vi "Registers in Data Clock.vi"(0 "register instruction":T6, 5 "config.resources":T4, 7 "time.resources":T3) -> (4 "read completion out":T5, 14 "ready for input":bool)   [LabVIEW 2020]
doc: "Sets/gets the configuration values for the instrument design libraries by connecting them to the Register Bus in the data clock domain.\n\n<B>Input Parameters</B>\n\n<B>register instruction</B> is the register bus instruction to execute.\n\n<B>config.resources</B> are references to the configuration registers.\n\n<B>Output Parameters</B>\n\n<B>read completion out</B> is the output of the last executed register instruction.\n\n<B>ready for input</B> is a flow control signal that indicates whether the Registers VI is ready to accept a new instruction."
uses:
  <instrlib>/_niInstr/Register Bus/v1/FPGA/Public/Register Instruction.ctl
  <instrlib>/_niInstr/Register Bus/v1/FPGA/Public/Read Completion.ctl
  <instrlib>/niUsrpRio/Time/v1/FPGA/Private/Time Resources.ctl
  <instrlib>/niUsrpRio/Time/v1/FPGA/Private/Future Event Resources.ctl
  <instrlib>/niUsrpRio/Config/v1/Shared/Subsystem ID.ctl
  <instrlib>/_niInstr/Register Bus/v1/FPGA/Private/Mux/Read Completion Mux (5 inputs).vi
  <instrlib>/_niInstr/Register Bus/v1/FPGA/niInstr Register Bus v1 FPGA.lvlib
  <instrlib>/niUsrpRio/Config/v1/FPGA/niUsrpRio Config v1 FPGA.lvlib
  <instrlib>/niUsrpRio/Config/v1/Shared/niUsrpRio Config v1 Shared.lvlib
  <instrlib>/niUsrpRio/Instruction Synchronizer/v1/FPGA/niUsrpRio Instruction Synchronizer v1 FPGA.lvlib
  <instrlib>/niUsrpRio/Time/v1/FPGA/niUsrpRio Time v1 FPGA.lvlib
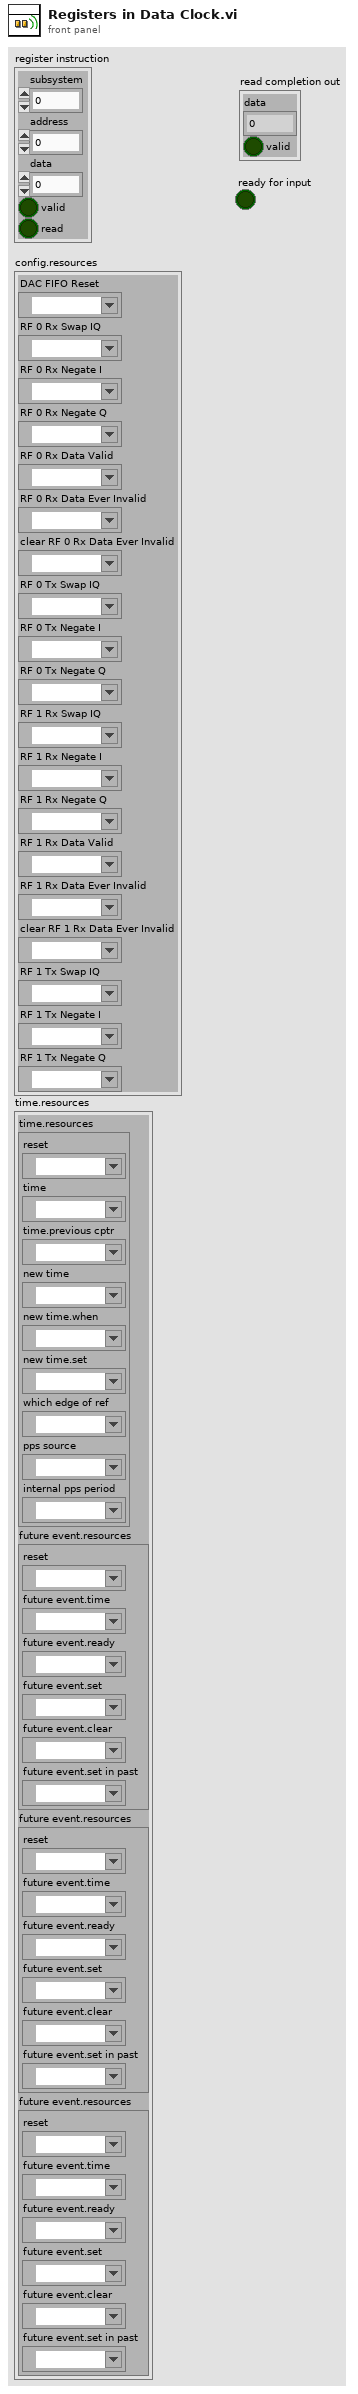
[diagram p1: front panel]
types:
  T1 = typedef "niUsrpRio Time v1 FPGA.lvlib/Time Resources.ctl" = cluster{"reset":refnum<k21>, "time":refnum<k21>, "time.previous cptr":refnum<k21>, "new time":refnum<k21>, "new time.when":refnum<k21>, "new time.set":refnum<k21>, "which edge of ref":refnum<k21>, "pps source":refnum<k21>, "internal pps period":refnum<k21>}
  T2 = typedef "niUsrpRio Time v1 FPGA.lvlib/Future Event Resources.ctl" = cluster{"reset":refnum<k21>, "future event.time":refnum<k21>, "future event.ready":refnum<k21>, "future event.set":refnum<k21>, "future event.clear":refnum<k21>, "future event.set in past":refnum<k21>}
  T3 = cluster{"time.resources":T1, "future event.resources":T2, "future event.resources":T2, "future event.resources":T2}
  T4 = cluster{"DAC FIFO Reset":refnum<k21>, "RF 0 Rx Swap IQ":refnum<k21>, "RF 0 Rx Negate I":refnum<k21>, "RF 0 Rx Negate Q":refnum<k21>, "RF 0 Rx Data Valid":refnum<k21>, "RF 0 Rx Data Ever Invalid":refnum<k21>, "clear RF 0 Rx Data Ever Invalid":refnum<k21>, "RF 0 Tx Swap IQ":refnum<k21>, "RF 0 Tx Negate I":refnum<k21>, "RF 0 Tx Negate Q":refnum<k21>, "RF 1 Rx Swap IQ":refnum<k21>, "RF 1 Rx Negate I":refnum<k21>, "RF 1 Rx Negate Q":refnum<k21>, "RF 1 Rx Data Valid":refnum<k21>, "RF 1 Rx Data Ever Invalid":refnum<k21>, "clear RF 1 Rx Data Ever Invalid":refnum<k21>, "RF 1 Tx Swap IQ":refnum<k21>, "RF 1 Tx Negate I":refnum<k21>, "RF 1 Tx Negate Q":refnum<k21>}
  T5 = typedef "niInstr Register Bus v1 FPGA.lvlib/Read Completion.ctl" = cluster{"data":u32, "valid":bool}
  T6 = typedef "niInstr Register Bus v1 FPGA.lvlib/Register Instruction.ctl" = cluster{"subsystem":u8, "address":u16, "data":u32, "valid":bool, "read":bool}
  T7 = typedef "niUsrpRio Config v1 Shared.lvlib/Subsystem ID.ctl" = enum8{"Identification", "Board Config", "Global Config", "Radio 0 Config", "Radio 1 Config", "Synchronization", "Time", "Future Events", "GPS", "Board Config (Data Clock)", "Instruction Synchronizer"}
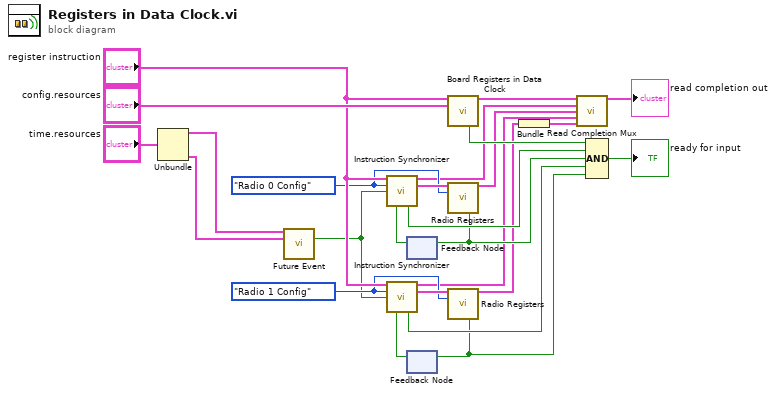
[diagram p0: block diagram]
diagram:
  w10 = Subsystem_ID."Radio 0 Config" ("Subsystem ID")
  w11 = Subsystem_ID."Radio 1 Config" ("Subsystem ID")
  n1 = Unbundle("time.resources") -> ("time.resources"=w8:T1, "future event.resources"=w7:T2)  [unwired: 2 out]
  n2 = call <instrlib>:"Future Event.vi"("time.resources"=w8, "future event.resources"=w7) -> ("event.occurred"=w6:bool)  [unwired: 12 in, 1 out]
  n3 = feedback #1() -> (w17:bool)  [unwired: 1 in]
  n4 = call <instrlib>:"Instruction Synchronizer.vi"("register instruction"="register instruction", "attached subsystem"=w10, "trigger"=w6, "ready for output"=w17) -> ("read completion out"=w5:T5, "register instruction out"=w18:T6, "ready for input"=w15:bool)  [unwired: 9 in]
  n5 = feedback #2() -> (w16:bool)  [unwired: 1 in]
  n6 = call <instrlib>:"Instruction Synchronizer.vi"("register instruction"="register instruction", "attached subsystem"=w11, "trigger"=w6, "ready for output"=w16) -> ("read completion out"=w3:T5, "register instruction out"=w20:T6, "ready for input"=w13:bool)  [unwired: 9 in]
  n7 = call <instrlib>:"Board Registers in Data Clock.vi"("register instruction"="register instruction", "resources"="config.resources") -> ("read completion"=w22:T5, "ready for input"=w21:bool)  [unwired: 12 in]
  n8 = call <instrlib>:"Radio Registers.vi"("register instruction"=w18, "Subsystem ID"=w10) -> ("read completion"=w4:T5, "ready for input"=w14:bool)  [unwired: 12 in]
  n9 = feedback-in #1(w14) -> ()
  n10 = call <instrlib>:"Radio Registers.vi"("register instruction"=w20, "Subsystem ID"=w11) -> ("read completion"=w1:T5, "ready for input"=w12:bool)  [unwired: 12 in]
  n11 = feedback-in #2(w12) -> ()
  n12 = Bundle("read completion"=w1) -> (w2:cluster{"read completion":T5})  [unwired: 1 in]
  n13 = call-poly <instrlib>:"Read Completion Mux.vi"("element 0"=w22, "element 1"=w5, "element 2"=w4, "element 3"=w3, "remaining elements (cluster)"=w2) -> ("read completion out"=→"read completion out":T5)  [unwired: 10 in]
  n14 = Compound Arithmetic op=AND(w21, w15, w14, w13, w12) -> (→"ready for input":bool)
